vi "Structure Selection and Quantization.vi"() -> ()   [LabVIEW 2023]
doc: "Demonstrates how different filter structures affect the characteristics of a fixed-point infinite impulse response (IIR) filter.\n\nComplete the following steps to use this VI.\n1) Run the VI.\n2) Observe the Magnitude Responses graph. This VI designs a floating-point Elliptic filter and displays the magnitude response of the filter.\n3) Specify a different structure in the <B>IIR Filter Implementation Structure</B> input. Notice that this change does not affect the magnitude response of the floating-point filter.\n4) Place a checkmark in the <B>Quantize the Filter</B> checkbox.\n5) Adjust the <B>Integer Word Length</B> values to ensure that the Quantized Filter plot approximates the Reference Filter plot in the Magnitude Responses graph. You also need to notice that no overflows or underflows occur in the Coefficients Report.\n6) Specify a different structure in the <B>IIR Filter Implementation Structure</B> input. Notice that the Quantized Filter plot changes because you changed the filter structure. You have to adjust the <B>Integer Word Length</B> values again to ensure that the Quantized Filter plot approximates the Reference Filter plot in the Magnitude Responses graph.\n7) Click the <B>STOP</B> button to stop this VI."
uses:
  <vilib>/addons/Digital Filter Design/_Objects.llb/DFD Quantization Sources.ctl
  <vilib>/addons/Digital Filter Design/_Objects.llb/DFD Quantization Settings.ctl
  <vilib>/addons/Digital Filter Design/FXPModel.llb/DFD FXP Quantize Coef (Advanced).vi
  <vilib>/addons/Digital Filter Design/Analysis.llb/DFD Plot Freq Response (Linear-Spaced).vi
  <vilib>/addons/Digital Filter Design/NI_DigFilterLicensed.lvlib
panel:
  in  "Tab Control":enum32{"Page 1"}(tab)
  in  "b/v iwl":i16 caption="Integer Word Length"
  in  "b/v wl":i16=16 caption="Word Length" min=1 max=32 step=1
  in  "a/k iwl":i16=2 caption="Integer Word Length"
  in  "a/k wl":i16=16 caption="Word Length" min=1 max=32 step=1
  in  "Quantization the Filter":bool
  in  "STOP":bool
  out "Coefficients Report":string
  out "Magnitude Responses":cluster{"f0":dbl, "df":dbl, "values":dbl[]}[](graph)
  out "Structure Diagram":u16(ring)
  in  "IIR Filter Implementation Structure":u16(ring) items=["Cascaded Second-Order Sections Form II", "Lattice ARMA (Basic Section)"]
  # "Quantizer Settings"
  # "Coefficients a/k"
  # "Coefficients b/v"
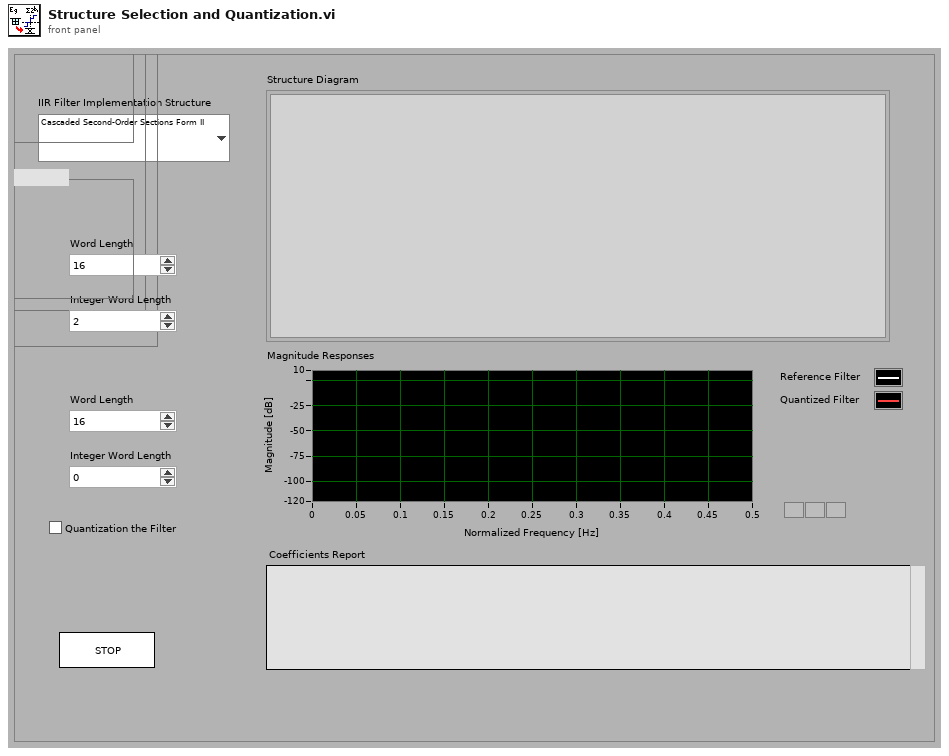
[diagram p1: front panel]
types:
  T1 = typedef "NI_DigFilterLicensed.lvlib/DFD Filter Obj.ctl" = cluster{"mSRate_Fs":dbl, "mSRate_Version":string, "mSRate_Comments":string, "mSRate_OrgCoef":T2, "mSRate_CurCoef":T2, "mSRate_Quantized?":bool, "mSRate_QCoef":T2, "mSRate_QSettings":T4[], "mSRate_Order":i32, "mSRate_Scaling":cluster{"mSRate_ScaleByPowerOf2?":bool, "mSRate_ScaleType":T6}}
  T2 = typedef "NI_DigFilterLicensed.lvlib/DFD Filter Coef.ctl" = cluster{"type":T3, "gain":dbl, "coef a (k)":dbl[], "coef b (v)":dbl[]}
  T3 = typedef "NI_DigFilterLicensed.lvlib/DFD Filter Structure Type Selector.ctl" = enum16{"Undefined", "FIR Direct Form", "FIR Direct Form Transposed", "FIR Symmetric", "FIR Antisymmetric", "IIR Direct Form I", "IIR Direct Form I Transposed", "IIR Direct Form II", "IIR Direct Form II Transposed", "IIR Cascaded Second Order Sections Form I", "IIR Cascaded Second Order Sections Form I Transposed", "IIR Cascaded Second Order Sections Form II", "IIR Cascaded Second Order Sections Form II Transposed", "Lattice Allpass (basic sections)", "Lattice Allpass (one multiplier sections)", "Lattice Allpass (normalized sections)", "Lattice AR (basic sections)", "Lattice AR (one multiplier sections)", "Lattice AR (normalized sections)", "Lattice MA (minimum phase)", "Lattice MA (maximum phase)", "Lattice ARMA (basic sections)", "Lattice ARMA (one multiplier sections)", "Lattice ARMA (normalized sections)"}
  T4 = typedef "NI_DigFilterLicensed.lvlib/dfd_Internal Quantization Settings.ctl" = cluster{"source":T5, "wl":i16, "iwl":i16, "overflow mode":enum16{"Saturation", "Wrap"}, "rounding mode":enum16{"Nearest", "Truncation"}, "signed?":bool}
  T5 = typedef "NI_DigFilterLicensed.lvlib/dfd_Internal Quantization Srcs.ctl" = u16
  T6 = typedef "NI_DigFilterLicensed.lvlib/DFD Coef Norm Type.ctl" = enum16{"No Norm", "Time Domain 1-Norm", "Time Domain 2-Norm", "Time Domain Inf-Norm"}
  T7 = typedef "NI_DigFilterLicensed.lvlib/DFD Quantization Settings.ctl" = cluster{"source":T8, "wl":i16, "iwl":i16, "overflow mode":enum16{"Saturation", "Wrap"}, "rounding mode":enum16{"Nearest", "Truncation"}, "signed?":bool}
  T8 = typedef "NI_DigFilterLicensed.lvlib/DFD Quantization Sources.ctl" = u16
  T9 = cluster{"source":T8, "wl":i16, "iwl":i16, "overflow mode":enum16{"Saturation", "Wrap"}, "rounding mode":enum16{"Nearest", "Truncation"}, "signed?":bool}
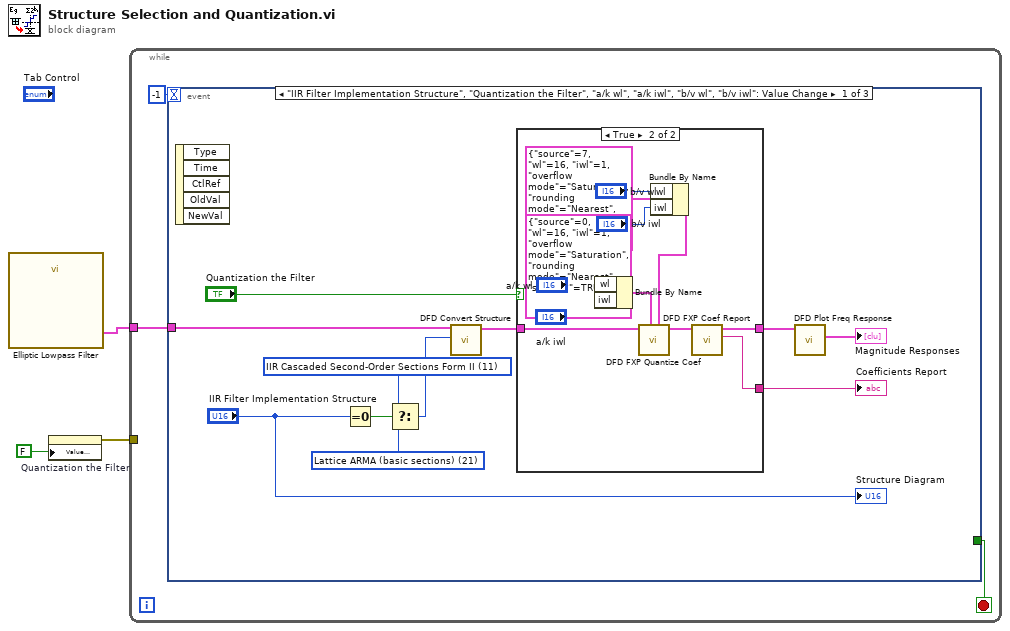
[diagram p0: block diagram]
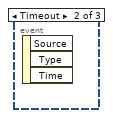
[diagram p3: hidden frame]
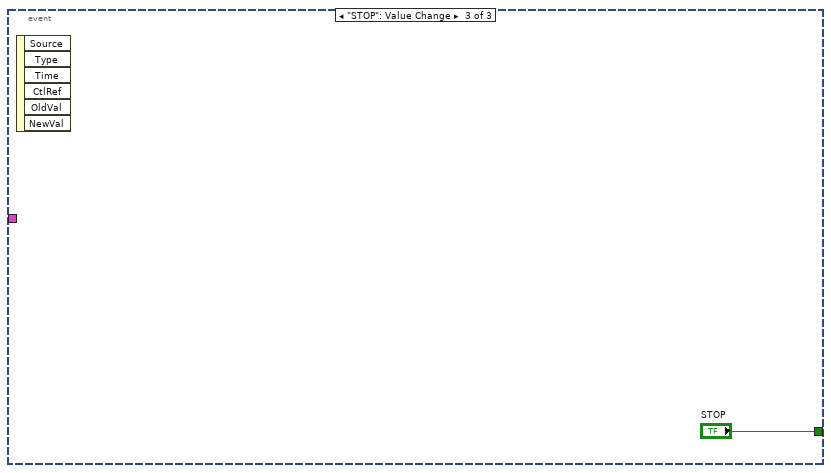
[diagram p4: hidden frame]
diagram:
  n1 = call "Elliptic Lowpass Filter"() -> ("filter out"=w1:T1)  [unwired: 1 in, 10 out]
  n2 = property on="Quantization the Filter" class="Bool (strict)"("Value (Signaling)"=FALSE) -> (error out=w3:errorcluster)  [unwired: 2 in, 1 out]
  n3 = while {
    tunnel: w1 -> [w6]
    tunnel: w3 -> [_]
    stop <- w4 stop-if-true
    n4 = event shown="[0] \"IIR Filter Implementation Structure\", \"Quantization the Filter\", \"a/k wl\", \"a/k iwl\", \"b/v wl\", \"b/v iwl\": Value Change" {
      selector: _ -> [_ _ _]
      dyn-events: _ -> [_ _ _]
      timeout: -1 -> [_ _ _]
      tunnel: w6 -> [w17 _ _]
      tunnel: [_ _ "STOP"] -> w4
      event "IIR Filter Implementation Structure", "Quantization the Filter", "a/k wl", "a/k iwl", "b/v wl", "b/v iwl": Value Change {
        w7 = u16 21 items=["FIR Direct Form"=1, "FIR Direct Form Transposed"=2, "FIR Symmetric"=3, "FIR Antisymmetric"=4, "IIR Direct Form I"=5, "IIR Direct Form I Transposed"=6, "IIR Direct Form II"=7, "IIR Direct Form II Transposed"=8, "IIR Cascaded Second-Order Sections Form I"=9, "IIR Cascaded Second-Order Sections Form I Transposed"=10, "IIR Cascaded Second-Order Sections Form II"=11, "IIR Cascaded Second-Order Sections Form II Transposed"=12, "Lattice Allpass (basic sections)"=13, "Lattice Allpass (one multiplier sections)"=14, "Lattice Allpass (normalized sections)"=15, "Lattice AR (basic sections)"=16, "Lattice AR (one multiplier sections)"=17, "Lattice AR (normalized sections)"=18, "Lattice MA (minimum phase)"=19, "Lattice MA (maximum phase)"=20, "Lattice ARMA (basic sections)"=21, "Lattice ARMA (one multiplier sections)"=22, "Lattice ARMA (normalized sections)"=23] ("target structure")
        w8 = u16 11 items=["FIR Direct Form"=1, "FIR Direct Form Transposed"=2, "FIR Symmetric"=3, "FIR Antisymmetric"=4, "IIR Direct Form I"=5, "IIR Direct Form I Transposed"=6, "IIR Direct Form II"=7, "IIR Direct Form II Transposed"=8, "IIR Cascaded Second-Order Sections Form I"=9, "IIR Cascaded Second-Order Sections Form I Transposed"=10, "IIR Cascaded Second-Order Sections Form II"=11, "IIR Cascaded Second-Order Sections Form II Transposed"=12, "Lattice Allpass (basic sections)"=13, "Lattice Allpass (one multiplier sections)"=14, "Lattice Allpass (normalized sections)"=15, "Lattice AR (basic sections)"=16, "Lattice AR (one multiplier sections)"=17, "Lattice AR (normalized sections)"=18, "Lattice MA (minimum phase)"=19, "Lattice MA (maximum phase)"=20, "Lattice ARMA (basic sections)"=21, "Lattice ARMA (one multiplier sections)"=22, "Lattice ARMA (normalized sections)"=23] ("target structure")
        n5 = event-data() -> ()  [unwired: 6 out]
        n6 = Equal To 0?(x="IIR Filter Implementation Structure") -> (x = 0?=w11:bool)
        n7 = Select(t=w8, s=w11, f=w7) -> (s? t:f=w10:u16)
        n8 = call <vilib>:"DFD Convert Structure.vi"("target structure"=w10, "filter in"=w17) -> ("filter out"=w12:T1)  [unwired: 1 in, 8 out]
        n9 = case shown="True" "Quantization the Filter" {
          tunnel: [_ w30] -> w16
          tunnel: [w18 w29] -> w14
          tunnel: w12 -> [w18 w28]
          frame False {
          }
          frame True {
            n10 = Bundle By Name(cluster=T9 {"source"=0, "wl"=16, "iwl"=1, "overflow mode"=enum."Saturation", "rounding mode"=enum."Nearest", "signed?"=TRUE} ("coefficients a/k quantizer"), "wl"="a/k wl", "iwl"="a/k iwl") -> (w23:T9)
            n11 = Bundle By Name(cluster=T7 {"source"=7, "wl"=16, "iwl"=1, "overflow mode"=enum."Saturation", "rounding mode"=enum."Nearest", "signed?"=TRUE} ("coefficients b/v quantizer"), "wl"="b/v wl", "iwl"="b/v iwl") -> (w19:T7)
            n12 = call-poly <vilib>:"DFD FXP Quantize Coef.vi"("coefficients b/v quantizer"=w19, "coefficients a/k quantizer"=w23, "filter in"=w28) -> ("filter out"=w27:T1)  [unwired: 2 in, 6 out]
            n13 = call <vilib>:"DFD FXP Coef Report.vi"("filter in"=w27) -> ("coefficients report"=w30:string, "filter out"=w29:T1)  [unwired: 1 in, 8 out]
          }
        }
        "Coefficients Report" <- w16
        n14 = call-poly <vilib>:"DFD Plot Freq Response.vi"("filter in"=w14) -> ("magnitude response"=→"Magnitude Responses":cluster{"f0":dbl, "df":dbl, "values":dbl[]}[])  [unwired: 7 in, 3 out]
        "Structure Diagram" <- "IIR Filter Implementation Structure"
      }
      event Timeout {
        n15 = event-data() -> ()  [unwired: 4 out]
      }
      event "STOP": Value Change {
        n16 = event-data() -> ()  [unwired: 7 out]
      }
    }
  }
